vi "Day 3 task 1 Alternate.vi"() -> ()   [LabVIEW 2022 SP3]
uses:
  <vilib>/regexp/Match Regular Expression.xnode
panel:
  out "Array":cluster{i32, i32}[][](array[cluster])
  out "sum":i64
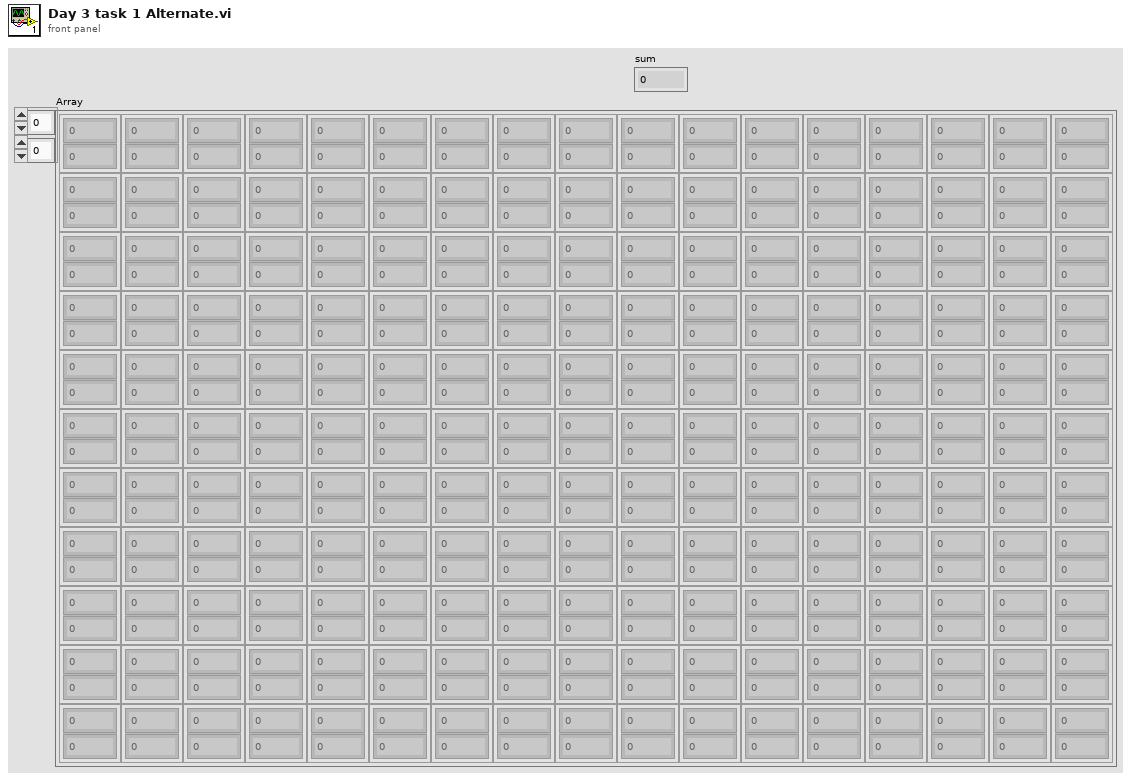
[diagram p1: front panel]
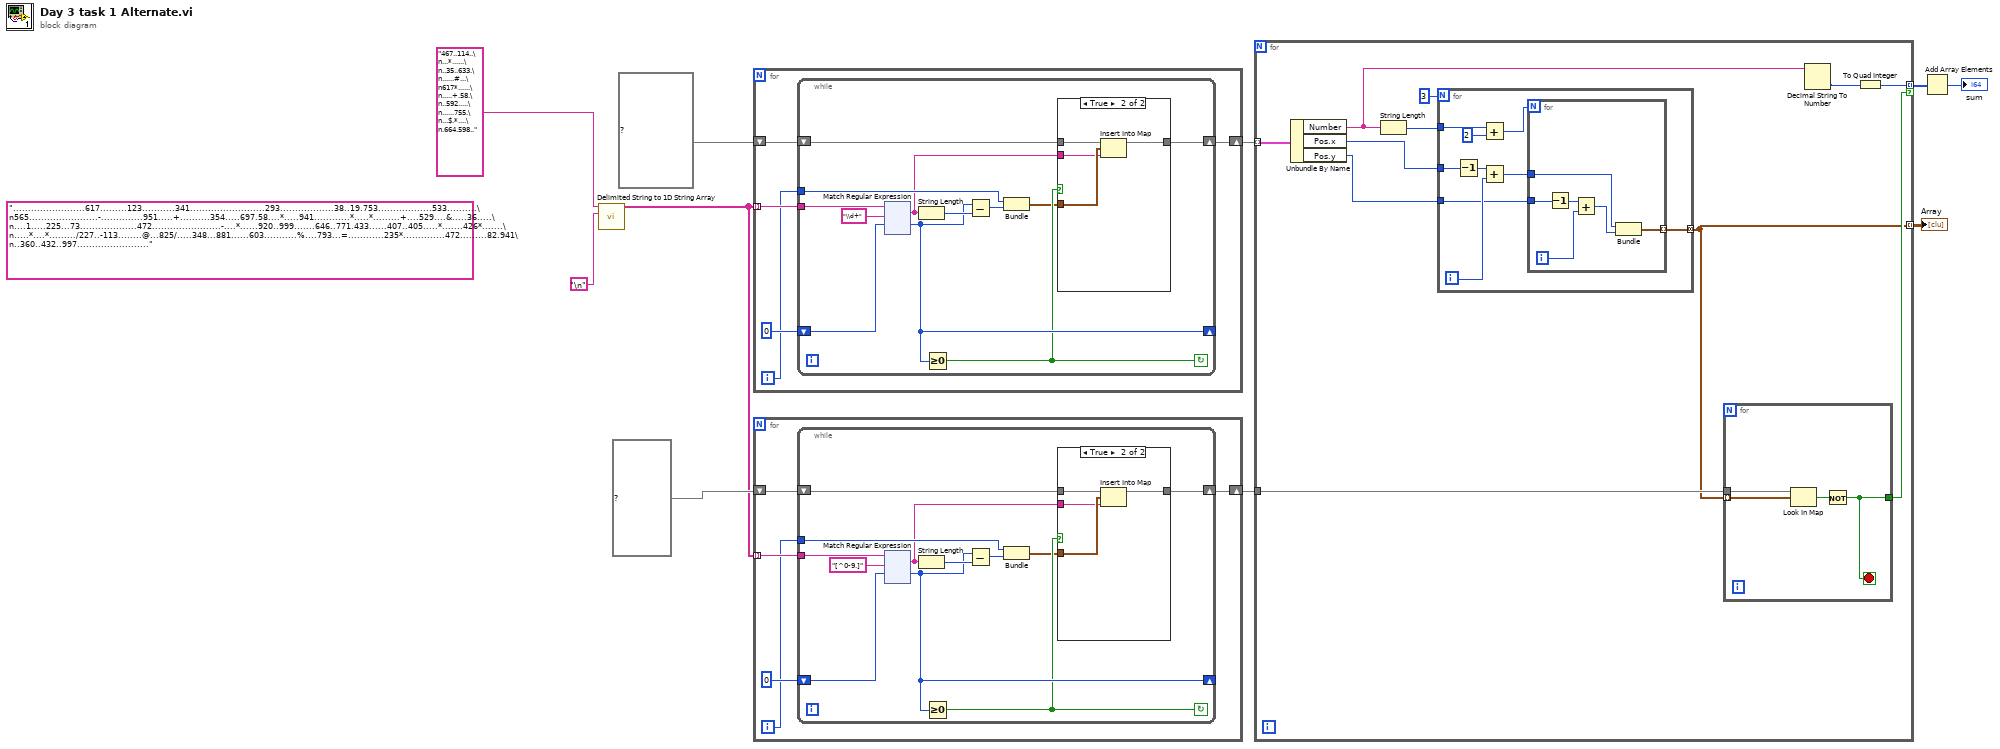
[diagram p0: block diagram]
diagram:
  (unwired) "........................617.........123...........341.........................293..................38..19.753..................533..........\n565.......................-..............951.....+..........354.....697.58....*.....941............*.....*.........+....529....&.....36.....\n....1.....225...73...................472.......................-....*......920..999.......646..771.433......407..405.....*.......426*.......\n.....*....*........./227..-113........@...825/.....348...881......603...........%....793...=............235*..............472.........82.941\n..360..432..997....................................*.....=............62...702......*..............................273..................*...\n...........&.......833.489.......@.........176...895............503.......$.......493...............929...............*.302....492.526......"
  n1 = call <vilib>:"Delimited String to 1D String Array.vi"("delimiter"="\n", "delimited string"="467..114..\n...*......\n..35..633.\n......#...\n617*......\n.....+.58.\n..592.....\n......755.\n...$.*....\n.664.598..") -> ("string array"=w7:string[])  [unwired: 9 in]
  n2 = for {
    tunnel: w7 -> [w14] mode=indexing
    shift-right: [w11] -> w6
    shift-left: map{cluster{"x":i32, "y":i32}, string} {} ("map in") -> [w15]
    i -> [w12]
    n3 = while {
      shift-right: [w18] -> w11
      shift-left: w15 -> [w19]
      tunnel: w14 -> [w26]
      shift-right: [w23] -> _
      shift-left: 0 -> [w27]
      tunnel: w12 -> [w21]
      stop <- w20 continue-if-true
      n4 = xnode "Match Regular Expression"("input string"=w26, "regular expression"="\\d+", "offset (0)"=w27) -> ("whole match"=w16:string, "offset past match"=w23:i32)  [unwired: 3 in, 3 out]
      n5 = String Length(string=w16) -> (length=w24:i32)
      n6 = Greater Or Equal To 0?(x=w23) -> (x >= 0?=w20:bool)
      n7 = Subtract(x=w23, y=w24) -> (x-y=w22:i32)
      n8 = Bundle(w21, w22) -> (w17:cluster{i32, i32})  [unwired: 1 in]
      n9 = case shown="True" w20 {
        tunnel: w19 -> [w28 w32]
        tunnel: [w28 w31] -> w18
        tunnel: w17 -> [_ w30]
        tunnel: w16 -> [_ w29]
        frame False {
        }
        frame True {
          n10 = Insert Into Map(map in=w32, key=w30, value=w29) -> (map out=w31:map{cluster{"x":i32, "y":i32}, string})  [unwired: 2 out]
        }
      }
    }
  }
  n11 = for {
    tunnel: w7 -> [w153] mode=indexing
    shift-right: [w150] -> w5
    shift-left: map{cluster{"x":i32, "y":i32}, string} {} ("map in") -> [w154]
    i -> [w151]
    n12 = while {
      shift-right: [w157] -> w150
      shift-left: w154 -> [w158]
      tunnel: w153 -> [w165]
      shift-right: [w162] -> _
      shift-left: 0 -> [w166]
      tunnel: w151 -> [w160]
      stop <- w159 continue-if-true
      n13 = xnode "Match Regular Expression"("input string"=w165, "regular expression"="[^0-9.]", "offset (0)"=w166) -> ("whole match"=w155:string, "offset past match"=w162:i32)  [unwired: 3 in, 3 out]
      n14 = String Length(string=w155) -> (length=w163:i32)
      n15 = Greater Or Equal To 0?(x=w162) -> (x >= 0?=w159:bool)
      n16 = Subtract(x=w162, y=w163) -> (x-y=w161:i32)
      n17 = Bundle(w160, w161) -> (w156:cluster{i32, i32})  [unwired: 1 in]
      n18 = case shown="True" w159 {
        tunnel: w158 -> [w167 w171]
        tunnel: [w167 w170] -> w157
        tunnel: w156 -> [_ w169]
        tunnel: w155 -> [_ w168]
        frame False {
        }
        frame True {
          n19 = Insert Into Map(map in=w171, key=w169, value=w168) -> (map out=w170:map{cluster{"x":i32, "y":i32}, string})  [unwired: 2 out]
        }
      }
    }
  }
  n20 = for {
    tunnel: w6 -> [w299] mode=indexing
    tunnel: w5 -> [w294]
    tunnel: [w291] -> w4 mode=indexing if=w290
    tunnel: [w289] -> w1 mode=indexing
    n21 = Unbundle By Name(w299) -> ("Number"=w293:string, "Pos.x"=w296:i32, "Pos.y"=w295:i32)
    n22 = String Length(string=w293) -> (length=w297:i32)
    n23 = for {
      N: 3 -> [_]
      tunnel: w297 -> [w312]
      tunnel: w296 -> [w309]
      tunnel: w295 -> [w305]
      tunnel: [w304] -> w289 mode=concatenating
      i -> [w307]
      n24 = Decrement(x=w309) -> (x-1=w308:i32)
      n25 = Add(x=w312, y=2) -> (x+y=w310:i32)
      n26 = Add(x=w308, y=w307) -> (x+y=w306:i32)
      n27 = for {
        N: w310 -> [_]
        tunnel: w306 -> [w318]
        tunnel: w305 -> [w316]
        tunnel: [w313] -> w304 mode=indexing
        i -> [w315]
        n28 = Decrement(x=w316) -> (x-1=w317:i32)
        n29 = Add(x=w317, y=w315) -> (x+y=w314:i32)
        n30 = Bundle(w318, w314) -> (w313:cluster{i32, i32})  [unwired: 1 in]
      }
    }
    n31 = for {
      tunnel: w294 -> [w303]
      tunnel: w289 -> [w302] mode=indexing
      tunnel: [w300] -> w290
      stop <- w300 stop-if-true
      n32 = Look In Map(map=w303, key=w302) -> (key not found?=w301:bool)  [unwired: 1 in, 1 out]
      n33 = Not(x=w301) -> (.not. x?=w300:bool)
    }
    n34 = Decimal String To Number(string=w293) -> (number=w292:i32)  [unwired: 2 in, 1 out]
    n35 = To Quad Integer(1:w292) -> (0:w291:i64)
  }
  "Array" <- w1
  n36 = Add Array Elements(numeric array=w4) -> (sum=→"sum":i64)
